vi "报警方式处理模块.vi"(7 "未报警状态？":bool, 8 "VISA资源名称":refnum<visa-resource-name>, 9 "探头地址":u8, 10 "探头限值":dbl, 11 "报警方式 i":T1) -> (2 "值改变？":bool, 3 "报警方式 o":T1)   [LabVIEW 2017]
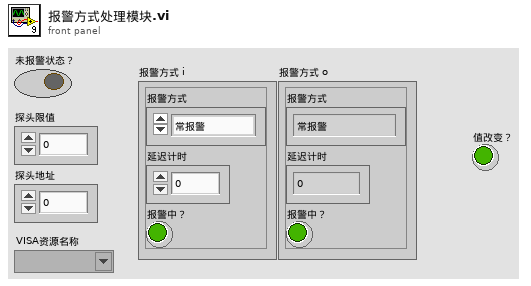
[diagram p1: front panel]
types:
  T1 = cluster{"报警方式":enum16{"常报警", "自动静音", "手动静音"}, "延迟计时":u16, "报警中？":bool}
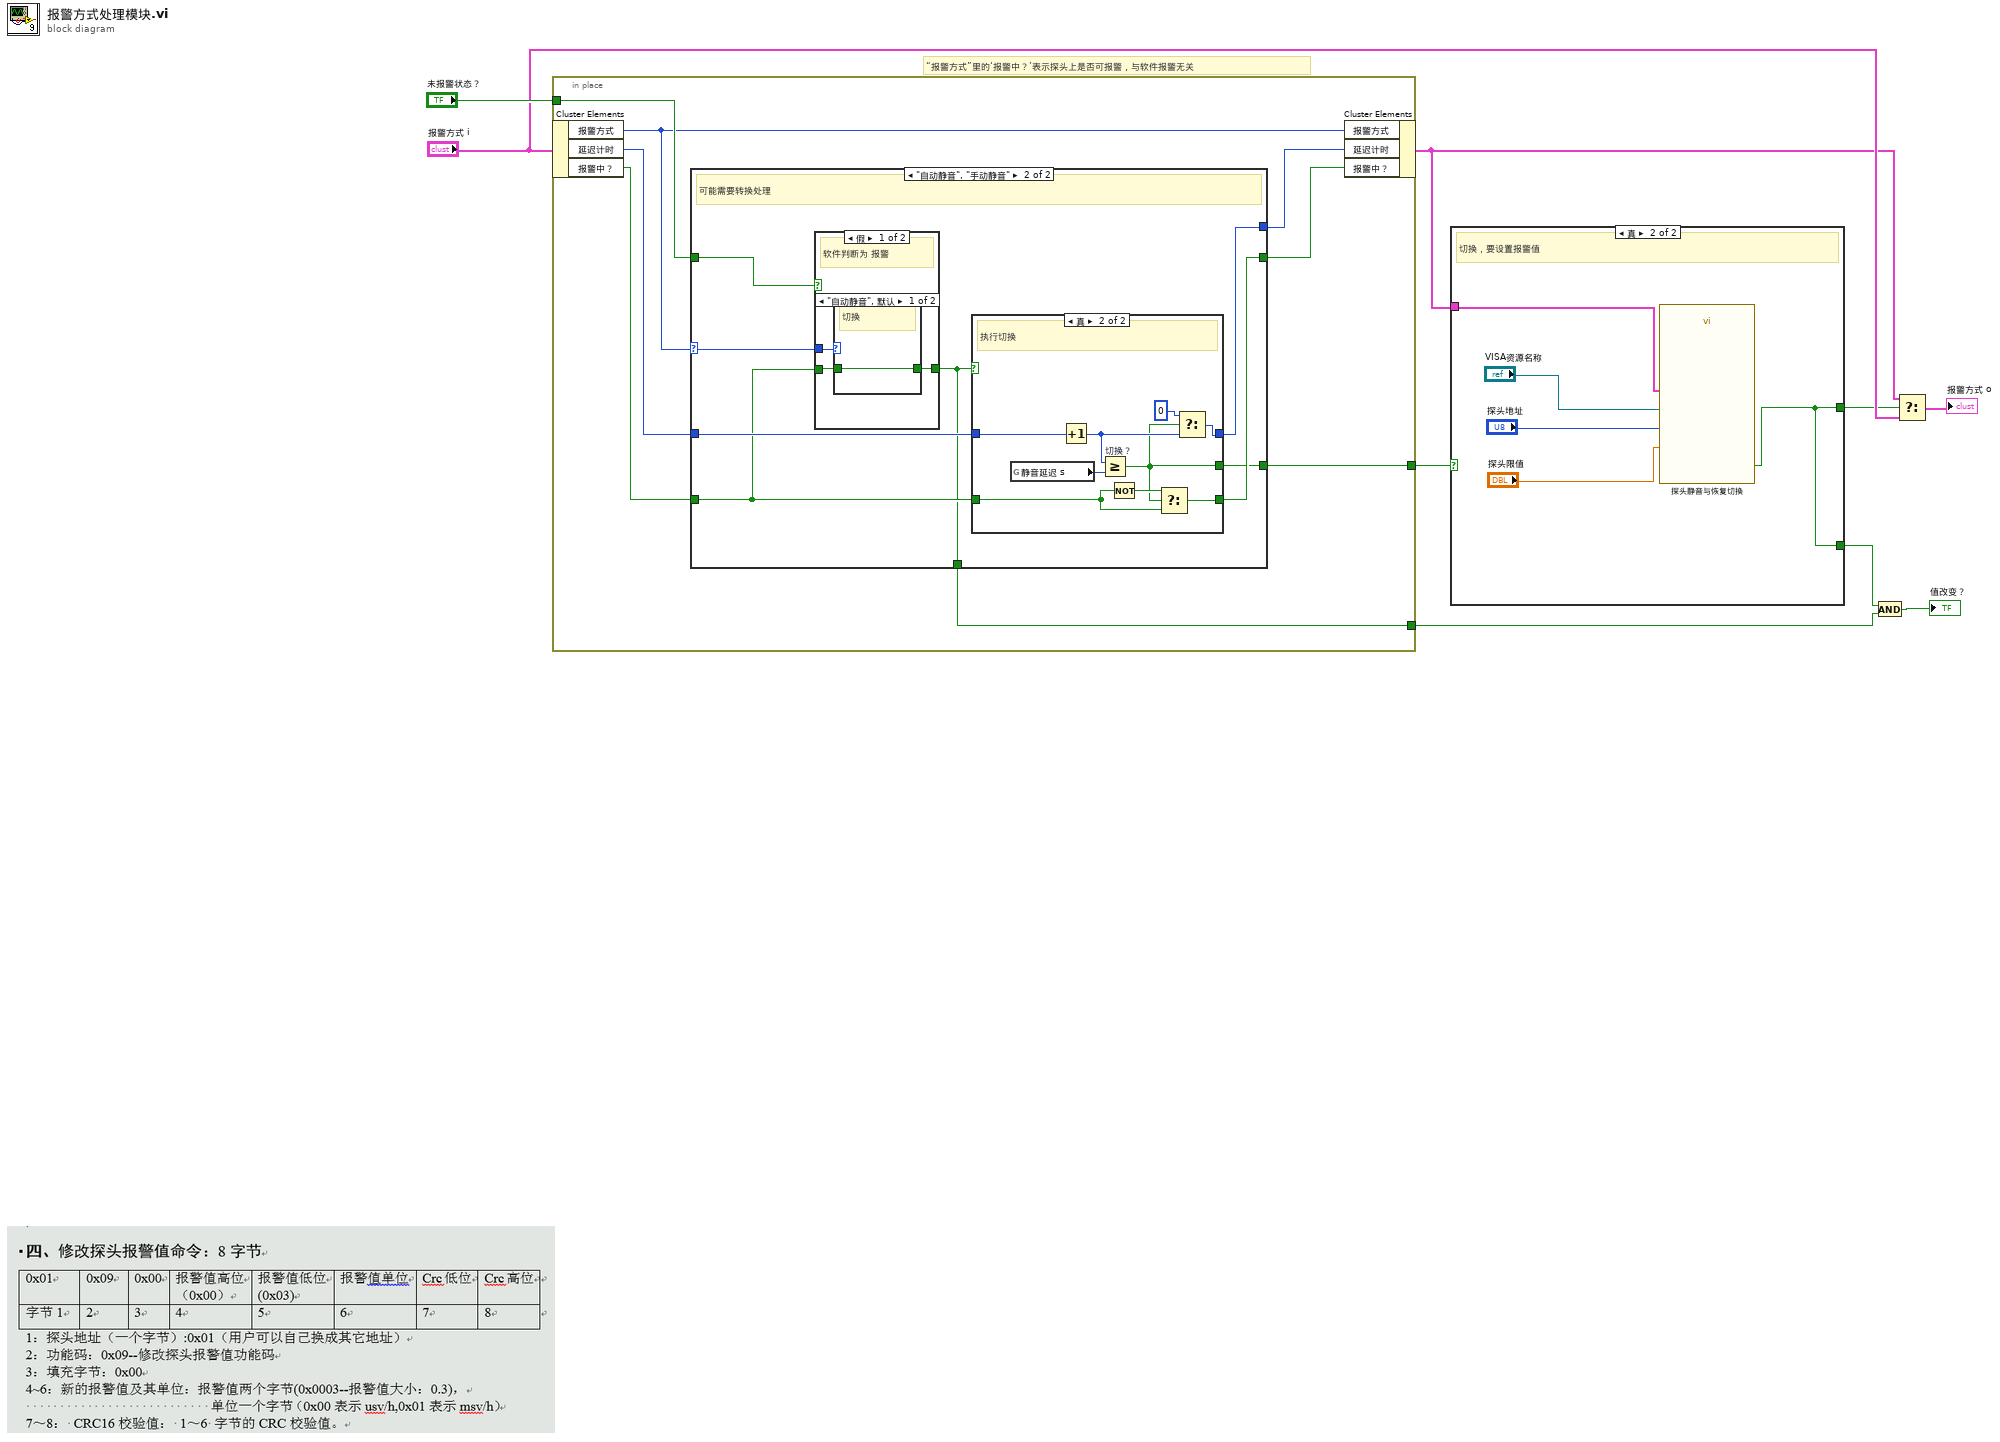
[diagram p0: block diagram]
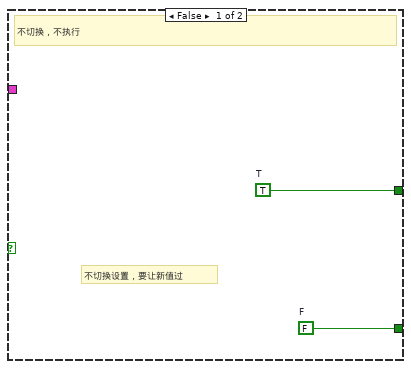
[diagram p2: hidden frame]
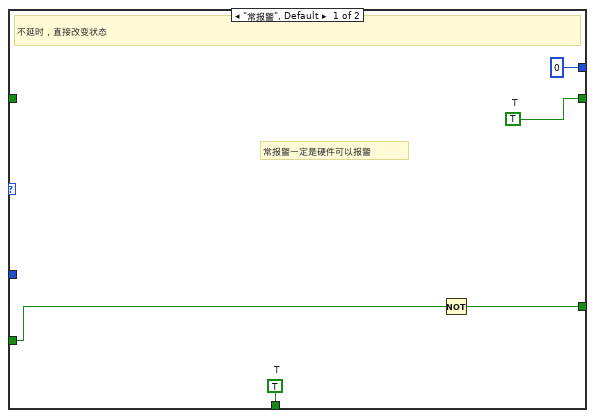
[diagram p3: hidden frame]
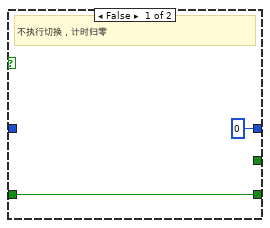
[diagram p4: hidden frame]
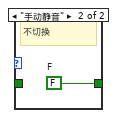
[diagram p5: hidden frame]
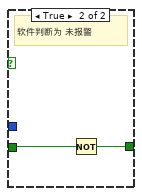
[diagram p6: hidden frame]
diagram:
  # "“报警方式”里的‘报警中？’表示探头上是否可报警，与软件报警无关"
  n1 = in-place {
    in-place-border: "未报警状态？" -> [w17]
    in-place-border: [w12] -> w8
    in-place-border: [w10] -> w4
    n2 = in-place-cluster #1("报警方式 i") -> ("报警方式"=w13:enum16{"常报警", "自动静音", "手动静音"}, "延迟计时"=w14:u16, "报警中？"=w16:bool)
    n3 = case shown="\"自动静音\", \"手动静音\"" w13 {
      selector: w13 -> [_ w29]
      tunnel: w17 -> [_ w30]
      tunnel: w16 -> [w19 w26]
      tunnel: [0 w27] -> w15
      tunnel: [w20 w25] -> w11
      tunnel: w14 -> [_ w28]
      tunnel: [w18 w24] -> w12
      tunnel: [w21 w23] -> w10
      frame "常报警", Default {
        w20 = TRUE  # T
        w21 = TRUE  # T
        # "常报警一定是硬件可以报警"
        # "不延时，直接改变状态"
        n4 = Not(x=w19) -> (.not. x?=w18:bool)
      }
      frame "自动静音", "手动静音" {
        # "可能需要转换处理"
        n5 = case shown="假" w30 {
          tunnel: w26 -> [w42 w48]
          tunnel: [w43 w47] -> w23
          tunnel: w29 -> [w44 _]
          frame False {
            # "软件判断为 报警"
            n6 = case shown="\"自动静音\", 默认" w44 {
              tunnel: [w45 w46] -> w43
              tunnel: w42 -> [w45 _]
              frame "自动静音", Default {
                # "切换"
              }
              frame "手动静音" {
                w46 = FALSE  # F
                # "不切换"
              }
            }
          }
          frame True {
            # "软件判断为 未报警"
            n7 = Not(x=w48) -> (.not. x?=w47:bool)
          }
        }
        n8 = case shown="真" w23 {
          tunnel: w28 -> [_ w39]
          tunnel: [0 w37] -> w27
          tunnel: w26 -> [w32 w36]
          tunnel: [w32 w34] -> w25
          tunnel: [_ w33] -> w24
          frame False {
            # "不执行切换，计时归零"
          }
          frame True {
            # "执行切换"
            n9 = global read "全局变量-35点监测.vi" "静音延迟 s"() -> (w40:u16)
            n10 = Increment(x=w39) -> (x+1=w38:u16)
            n11 = Greater Or Equal? "切换？"(x=w38, y=w40) -> (x >= y?=w33:bool)
            n12 = Not(x=w36) -> (.not. x?=w35:bool)
            n13 = Select(t=w35, s=w33, f=w36) -> (s? t:f=w34:bool)
            n14 = Select(t=0, s=w33, f=w38) -> (s? t:f=w37:i32)
          }
        }
      }
    }
    n15 = in-place-cluster #1("报警方式"=w13, "延迟计时"=w15, "报警中？"=w11) -> (w5:T1)
  }
  n16 = case shown="真" w8 {
    tunnel: [w50 w51] -> w3
    tunnel: w5 -> [_ w55]
    tunnel: [w49 w51] -> w1
    frame False {
      w49 = FALSE  # F
      w50 = TRUE  # T
      # "不切换设置，要让新值过"
      # "不切换，不执行"
    }
    frame True {
      # "切换，要设置报警值"
      n17 = call "探头静音与恢复切换.vi"("VISA资源名称"="VISA资源名称", "探头地址"="探头地址", "限值1"="探头限值", "切换至方式"=w55) -> ("切换成功？"=w51:bool)  [unwired: 7 in]
    }
  }
  n18 = And(x=w1, y=w4) -> (x .and. y?=→"值改变？":bool)
  n19 = Select(t=w5, s=w3, f="报警方式 i") -> (s? t:f=→"报警方式 o":T1)
